vi "Shutdown Process.vi"(8 "error in (no error)":errorcluster, 10 "Process Name":string, 11 "Application In":refnum<class "Application.lvclass">) -> (0 "error out":errorcluster, 3 "Application Out":refnum<class "Application.lvclass">)   [LabVIEW 2020, in "Application.lvclass"]
doc: "Stops and clears down a specific process owned by the application and removes it from the application."
uses:
  Application.lvclass
  C:/git/astemes-triarc-framework/source/Framework/Process/Process.lvclass
  Process/Process.lvclass/Process.ctl
  Application.lvclass/Application.ctl
  <vilib>/Utility/error.llb/Clear Errors.vi
  Process/Private/SubVIs/Handle Debug Data.vi
  Process/Private/SubVIs/Wait for finish.vi
  Process/Private/SubVIs/Set Lifecycle State.vi
  Logging/Log Debug.vi
  <vilib>/AdvancedString/1D String Array to Delimited String.vi
  <vilib>/Utility/High Resolution Relative Seconds.vi
  Process/Public/Read Name.vi
  <vilib>/Utility/error.llb/Error Cluster From Error Code.vi
  Callback/Callback.lvclass
  Process/Process.lvclass
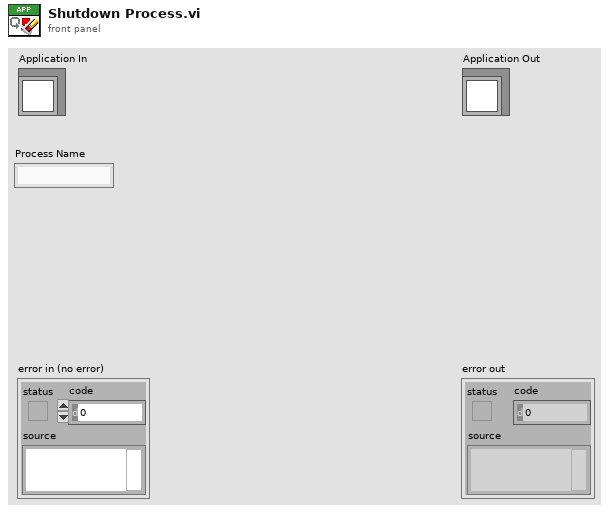
[diagram p1: front panel]
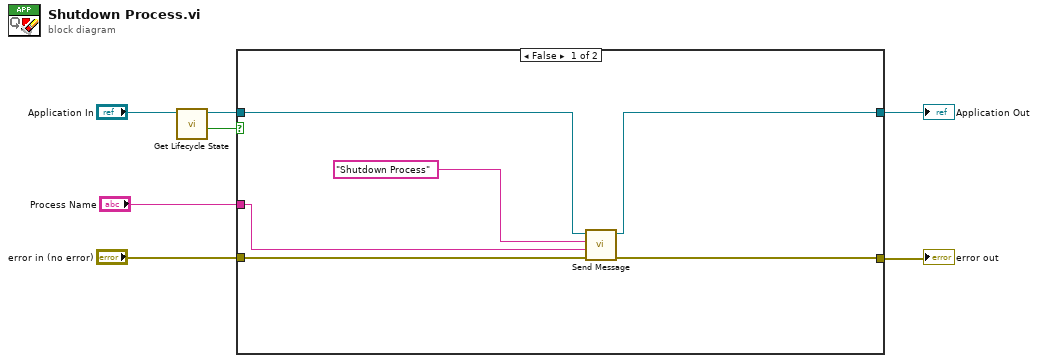
[diagram p0: block diagram]
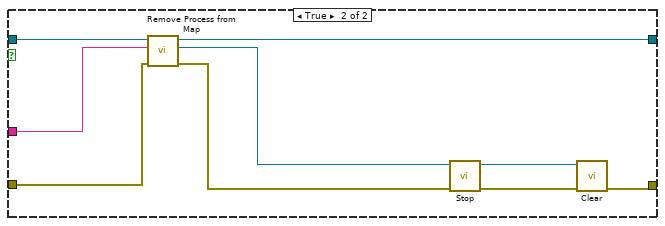
[diagram p2: hidden frame]
diagram:
  n1 = call "Get Lifecycle State.vi"("Process In"="Application In") -> ("In Process Loop?"=w2:bool, "Process Out"=w3:refnum<class "Application.lvclass">)  [unwired: 7 in, 2 out]
  n2 = case shown="False" w2 {
    tunnel: "error in (no error)" -> [w13 w18]
    tunnel: "Process Name" -> [w9 w15]
    tunnel: [w11 w14] -> w1
    tunnel: [w12 w21] -> w4
    tunnel: w3 -> [w10 w19]
    frame False {
      n3 = call "Send Message.vi"("error in (no error)"=w13, "Message Data"=w9, "Message"="Shutdown Process", "Process In"=w10) -> ("error out"=w12:errorcluster, "Process Out"=w11:refnum<class "Application.lvclass">)  [unwired: 6 in]
    }
    frame True {
      n4 = call "Remove Process from Map.vi"("error in (no error)"=w18, "Process Name"=w15, "Application In"=w19) -> ("error out"=w16:errorcluster, "Process"=w17:refnum<class "Process.lvclass">, "Application Out"=w14:refnum<class "Application.lvclass">)  [unwired: 6 in]
      n5 = call "Stop.vi"("error in (no error)"=w16, "Process In"=w17) -> ("error out"=w22:errorcluster, "Process Out"=w20:refnum<class "Process.lvclass">)  [unwired: 7 in, 1 out]
      n6 = call-dynamic "Clear.vi"("error in (no error)"=w22, "Process In"=w20) -> ("error out"=w21:errorcluster)  [unwired: 9 in]
    }
  }
  "error out" <- w4
  "Application Out" <- w1
